vi "PTSequencer.contents.vi"   [LabVIEW 2014, in "PTSequencer.lvlib"]
uses:
  PTSequencer.lvlib
panel:
  # "Refer to block diagram for details"
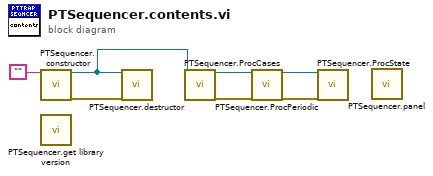
[diagram p0: block diagram]
diagram:
  n1 = call "PTSequencer.constructor.vi"("name"="") -> ("i ref out"=w6:refnum<vi>, "error out"=w7:errorcluster)  [unwired: 16 in, 1 out]
  n2 = call "PTSequencer.get library version.vi"() -> ()  [unwired: 1 in, 1 out]
  n3 = call "PTSequencer.destructor.vi"("i ref in"=w6, "error in (no error)"=w7) -> ()  [unwired: 17 in, 1 out]
  n4 = call "PTSequencer.ProcCases.vi"("i ref in"=w6) -> ("i ref out"=w5:refnum<vi>, "error out"=w3:errorcluster)  [unwired: 16 in, 1 out]
  n5 = call "PTSequencer.ProcPeriodic.vi"("i ref in"=w5, "error in (no error)"=w3) -> ("i ref out"=w4:refnum<vi>, "error out"=w2:errorcluster)  [unwired: 15 in, 1 out]
  n6 = call "PTSequencer.ProcState.vi"("i ref in"=w4, "error in"=w2) -> ()  [unwired: 15 in, 3 out]
  n7 = call "PTSequencer.panel.vi"() -> ()  [unwired: 20 in]
